vi "Car Wash Server.vi"() -> ()   [LabVIEW 2021]
uses:
  <vilib>/Utility/file.llb/Write Delimited Spreadsheet (string).vi
  <vilib>/Utility/file.llb/Read Delimited Spreadsheet (string).vi
panel:
  in  "Server Tab":enum32{"Page 1", "Page 2"}(tab)
  in  "Password":string
  in  "User Name":string
  in  "Login Button":bool
  out "Total Economy Wash":i32
  out "Total Deluxe Wash":i32
  out "Log Record":string[][](table)
  in  "Logout button":bool
  # "Server Login"
  # "Server"
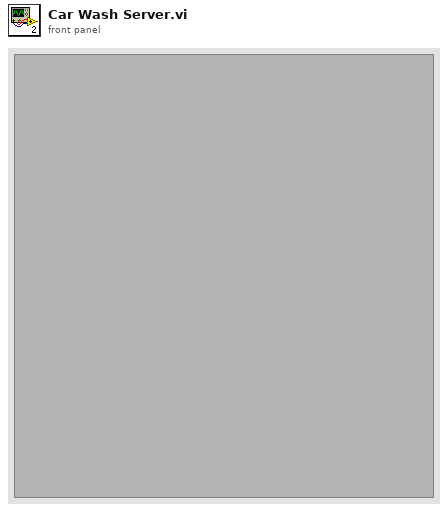
[diagram p1: front panel]
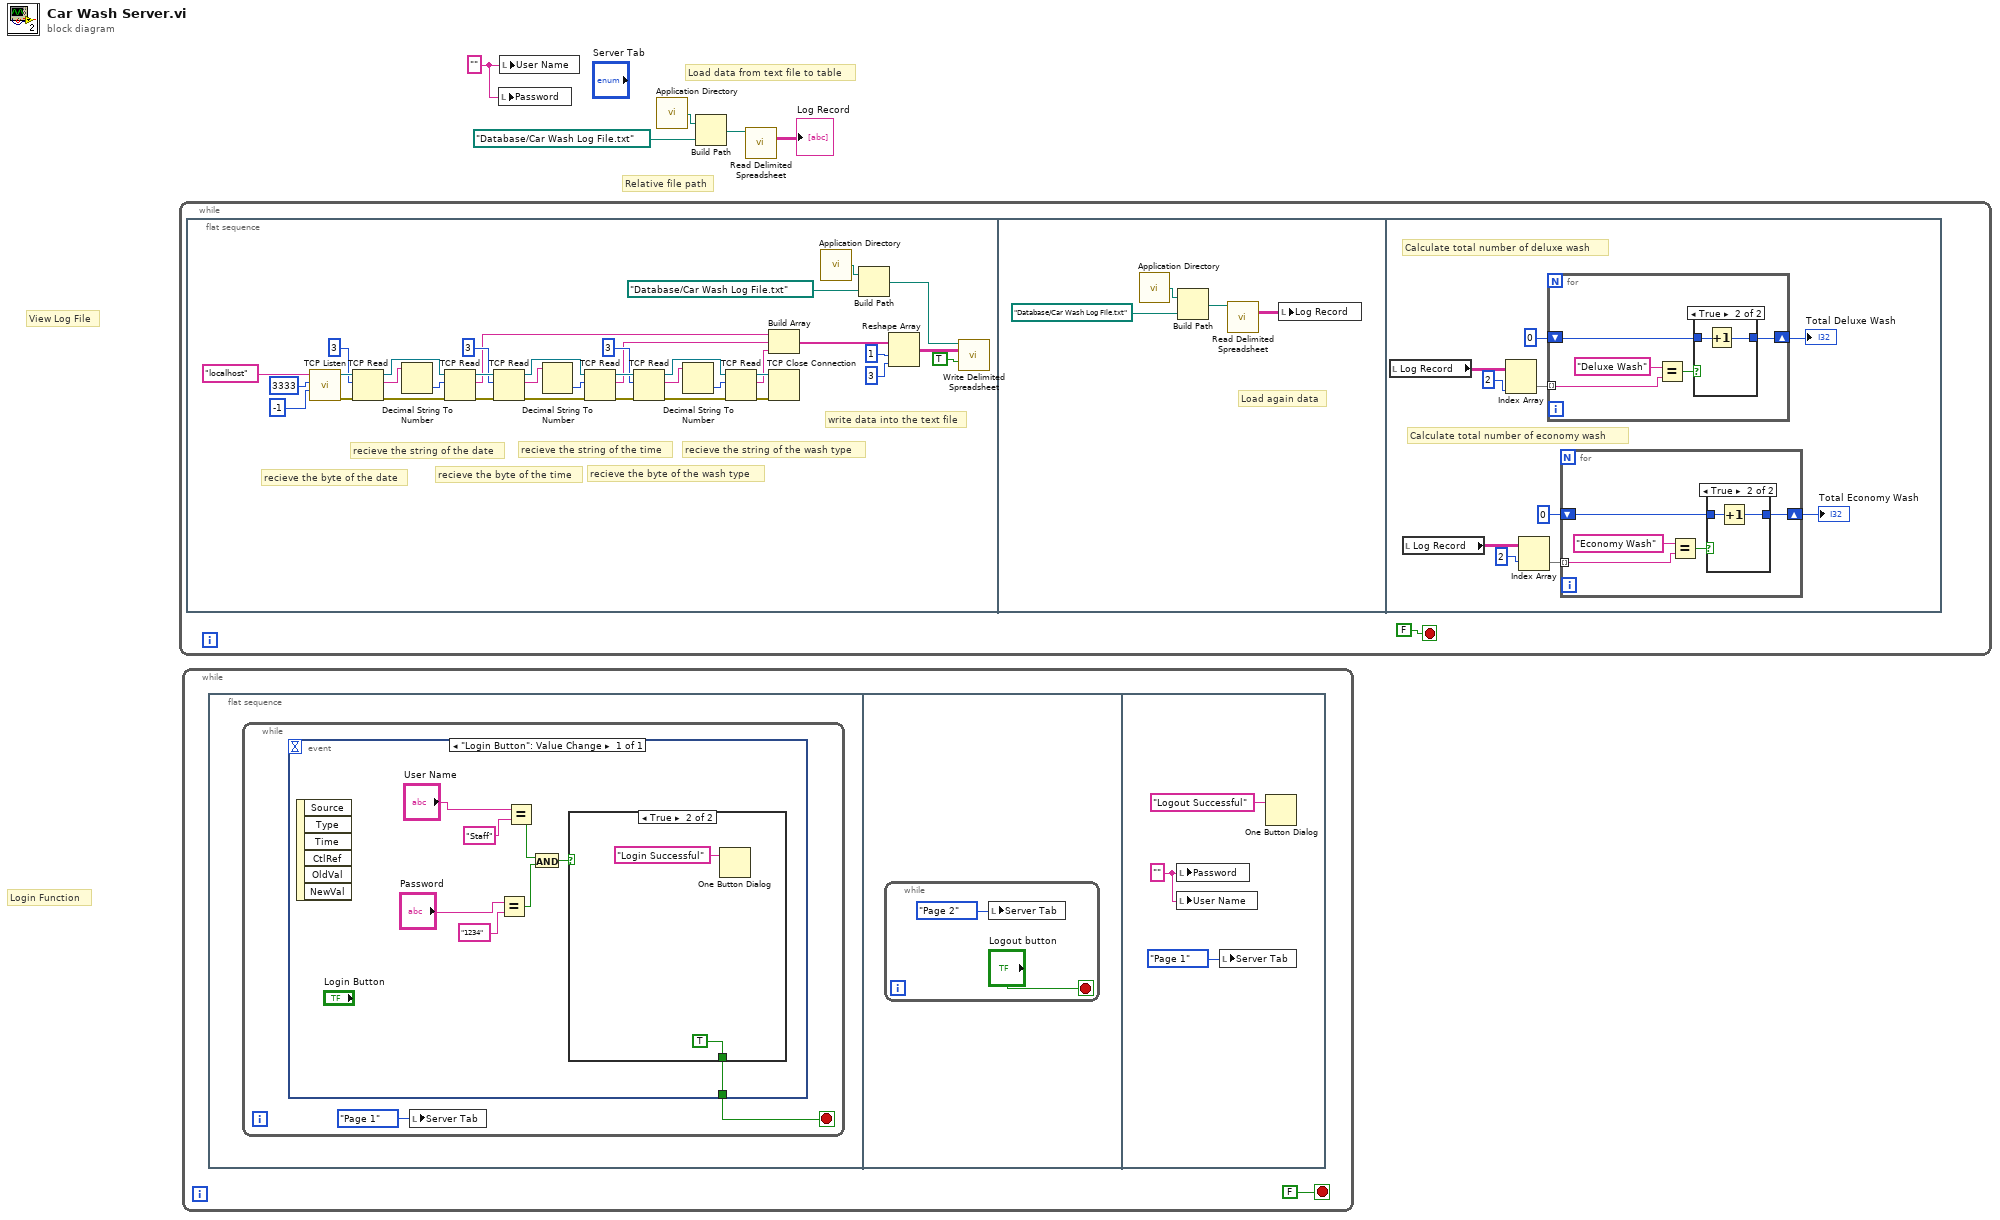
[diagram p0: block diagram]
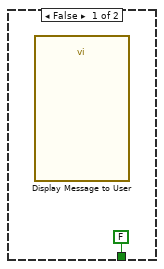
[diagram p2: hidden frame]
diagram:
  w1 = "" ("User Name")
  # "View Log File"
  # "Login Function"
  # "Relative file path"
  # "Load data from text file to table"
  n1 = while {
    stop <- FALSE stop-if-true
    n2 = flat-sequence {
      frame #0 {
        # "write data into the text file"
        # "recieve the string of the wash type"
        # "recieve the byte of the wash type"
        # "recieve the string of the time"
        # "recieve the byte of the time"
        # "recieve the string of the date"
        # "recieve the byte of the date"
        n3 = call <vilib>:"TCP Listen.vi"("timeout ms (wait forever: -1)"=-1, "port"=u16 3333, "service name"="localhost") -> ("error out"=w38:errorcluster, "connection ID"=w37:refnum<k5>)  [unwired: 4 in, 3 out]
        n4 = TCP Read(connection ID=w37, bytes to read=3, error in (no error)=w38) -> (connection ID out=w36:refnum<k5>, data out=w23:string, error out=w35:errorcluster)  [unwired: 2 in]
        n5 = Decimal String To Number(string=w23) -> (number=w22:i32)  [unwired: 2 in, 1 out]
        n6 = TCP Read(connection ID=w36, bytes to read=w22, error in (no error)=w35) -> (connection ID out=w34:refnum<k5>, data out=w17:string, error out=w33:errorcluster)  [unwired: 2 in]
        n7 = TCP Read(connection ID=w34, bytes to read=3, error in (no error)=w33) -> (connection ID out=w39:refnum<k5>, data out=w21:string, error out=w40:errorcluster)  [unwired: 2 in]
        n8 = Decimal String To Number(string=w21) -> (number=w20:i32)  [unwired: 2 in, 1 out]
        n9 = TCP Read(connection ID=w39, bytes to read=w20, error in (no error)=w40) -> (connection ID out=w32:refnum<k5>, data out=w16:string, error out=w31:errorcluster)  [unwired: 2 in]
        n10 = TCP Read(connection ID=w32, bytes to read=3, error in (no error)=w31) -> (connection ID out=w30:refnum<k5>, data out=w19:string, error out=w29:errorcluster)  [unwired: 2 in]
        n11 = Decimal String To Number(string=w19) -> (number=w18:i32)  [unwired: 2 in, 1 out]
        n12 = TCP Read(connection ID=w30, bytes to read=w18, error in (no error)=w29) -> (connection ID out=w28:refnum<k5>, data out=w15:string, error out=w27:errorcluster)  [unwired: 2 in]
        n13 = Build Array "Build Array"(w17, w16, w15) -> (w14:string[])
        n14 = TCP Close Connection(connection ID=w28, error in (no error)=w27) -> ()  [unwired: 1 in, 2 out]
        n15 = call <vilib>:"Application Directory.vi"() -> ("Application Directory"=w11:path)
        n16 = Build Path(base path=w11, name or relative path=path "Database/Car Wash Log File.txt") -> (appended path=w8:path)
        n17 = Reshape Array(w14, 1 ("dimension size"), 3 ("dimension size")) -> (w7:string[][])
        n18 = call-poly <vilib>:"Write Delimited Spreadsheet.vi"("file path (dialog if empty)"=w8, "2D data"=w7, "append to file? (new file:F)"=TRUE) -> ()  [unwired: 11 in, 2 out]
      }
      frame #1 {
        # "Load again data"
        n19 = call <vilib>:"Application Directory.vi"() -> ("Application Directory"=w46:path)
        n20 = Build Path(base path=w46, name or relative path=path "Database/Car Wash Log File.txt") -> (appended path=w47:path)
        n21 = call-poly <vilib>:"Read Delimited Spreadsheet.vi"("file path (dialog if empty)"=w47) -> ("all rows"=w44:string[][])  [unwired: 9 in, 5 out]
        n22 = local write "Log Record"(w44) -> ()
      }
      frame #2 {
        # "Calculate total number of economy wash"
        # "Calculate total number of deluxe wash"
        n23 = local read "Log Record"() -> (w52:string[][])
        n24 = local read "Log Record"() -> (w57:string[][])
        n25 = Index Array(array=w52, index (col)=2 ("disabled index (col)")) -> (element=w53:string[])  [unwired: 1 in]
        n26 = Index Array(array=w57, index (col)=2 ("disabled index (col)")) -> (element=w56:string[])  [unwired: 1 in]
        n27 = for {
          shift-right: [w69] -> w54
          shift-left: 0 -> [w70]
          tunnel: w53 -> [w66] mode=indexing
          n28 = Equal?(x="Deluxe Wash", y=w66) -> (x = y?=w67:bool)
          n29 = case shown="True" w67 {
            tunnel: w70 -> [w71 w73]
            tunnel: [w71 w72] -> w69
            frame False {
            }
            frame True {
              n30 = Increment(x=w73) -> (x+1=w72:i32)
            }
          }
        }
        "Total Deluxe Wash" <- w54
        n31 = for {
          shift-right: [w61] -> w55
          shift-left: 0 -> [w62]
          tunnel: w56 -> [w58] mode=indexing
          n32 = Equal?(x="Economy Wash", y=w58) -> (x = y?=w59:bool)
          n33 = case shown="True" w59 {
            tunnel: w62 -> [w63 w65]
            tunnel: [w63 w64] -> w61
            frame False {
            }
            frame True {
              n34 = Increment(x=w65) -> (x+1=w64:i32)
            }
          }
        }
        "Total Economy Wash" <- w55
      }
    }
  }
  n35 = while {
    stop <- FALSE stop-if-true
    n36 = flat-sequence {
      frame #0 {
        n37 = while {
          stop <- w76 stop-if-true
          n38 = event shown="[0] \"Login Button\": Value Change" {
            selector: _ -> [_]
            dyn-events: _ -> [_]
            timeout: _ -> [_]
            tunnel: [w82] -> w76
            event "Login Button": Value Change {
              n39 = event-data() -> ()  [unwired: 1 in, 6 out]
              n40 = Equal?(x="Password", y="1234") -> (x = y?=w79:bool)
              n41 = Equal?(x="User Name", y="Staff") -> (x = y?=w80:bool)
              n42 = And(x=w80, y=w79) -> (x .and. y?=w81:bool)
              n43 = case shown="True" w81 {
                tunnel: [FALSE TRUE] -> w82
                frame False {
                  n44 = call "Display Message to User"() -> ()  [unwired: 10 in, 2 out]
                }
                frame True {
                  n45 = One Button Dialog(message="Login Successful") -> ()  [unwired: 1 in, 1 out]
                }
              }
            }
          }
          n46 = local write "Server Tab"(enum32{"Page 1", "Page 2"}."Page 1" ("Server Tab")) -> ()
        }
      }
      frame #1 {
        n47 = while {
          stop <- "Logout button" stop-if-true
          n48 = local write "Server Tab"(enum32{"Page 1", "Page 2"}."Page 2" ("Server Tab")) -> ()
        }
      }
      frame #2 {
        w91 = "" ("User Name")
        n49 = local write "Password"(w91) -> ()
        n50 = local write "User Name"(w91) -> ()
        n51 = local write "Server Tab"(enum32{"Page 1", "Page 2"}."Page 1" ("Server Tab")) -> ()
        n52 = One Button Dialog(message="Logout Successful") -> ()  [unwired: 1 in, 1 out]
      }
    }
  }
  n53 = local write "Password"(w1) -> ()
  n54 = local write "User Name"(w1) -> ()
  n55 = call <vilib>:"Application Directory.vi"() -> ("Application Directory"=w3:path)
  n56 = Build Path(base path=w3, name or relative path=path "Database/Car Wash Log File.txt") -> (appended path=w2:path)
  n57 = call-poly <vilib>:"Read Delimited Spreadsheet.vi"("file path (dialog if empty)"=w2) -> ("all rows"=→"Log Record":string[][])  [unwired: 9 in, 5 out]
